vi "updateMinMax.vi"(8 "error in (no error)":errorcluster, 11 "PIDController in":refnum<class "PIDController.lvclass">) -> (0 "error out":errorcluster, 3 "PIDController out":refnum<class "PIDController.lvclass">)   [LabVIEW 2025, in "PIDController.lvclass"]
uses:
  PIDController.lvclass
  PIDController.lvclass/PIDController.ctl
panel:
  in  "a_max":dbl
  in  "a_min":dbl
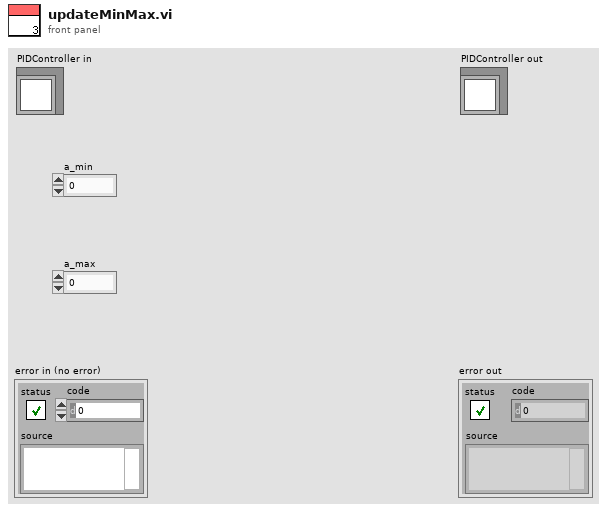
[diagram p1: front panel]
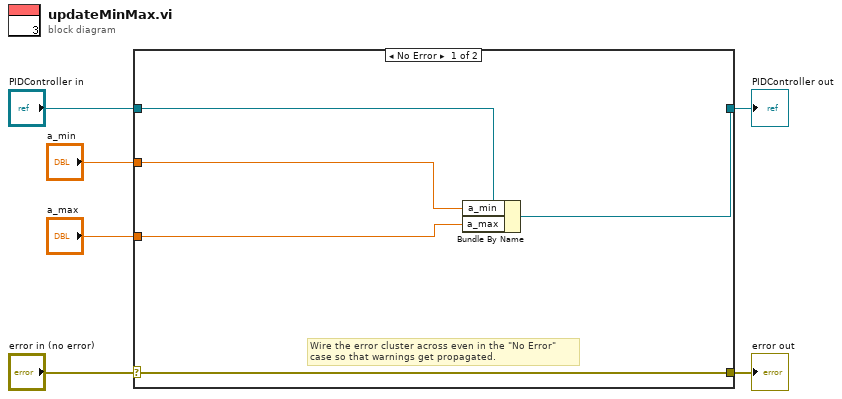
[diagram p0: block diagram]
diagram:
  n1 = case shown="No Error" "error in (no error)" {
    selector: "error in (no error)" -> [w11 w13]
    tunnel: [w11 w13] -> w5
    tunnel: [w9 w12] -> w3
    tunnel: "PIDController in" -> [w10 w12]
    tunnel: "a_min" -> [w8 _]
    tunnel: "a_max" -> [w7 _]
    frame No Error {
      # "Wire the error cluster across even in the \"No Error\"\ncase so that warnings get propagated."
      n2 = Bundle By Name(cluster=w10, "a_min"=w8, "a_max"=w7) -> (w9:refnum<class "PIDController.lvclass">)
    }
    frame Error {
    }
  }
  "error out" <- w5
  "PIDController out" <- w3
